vi "JsonTesting.vi"() -> ()   [LabVIEW 2012]
uses:
  <vilib>/httpClient/LabVIEWHTTPClient.lvlib
  <vilib>/LVH/i3 JSON/i3-json.lvlib
panel:
  out "body 3":string
  out "Tree 3":string(tree)
  out "body 2":string
  out "Tree 2":string(tree)
  out "Tree":string(tree)
  out "body":string
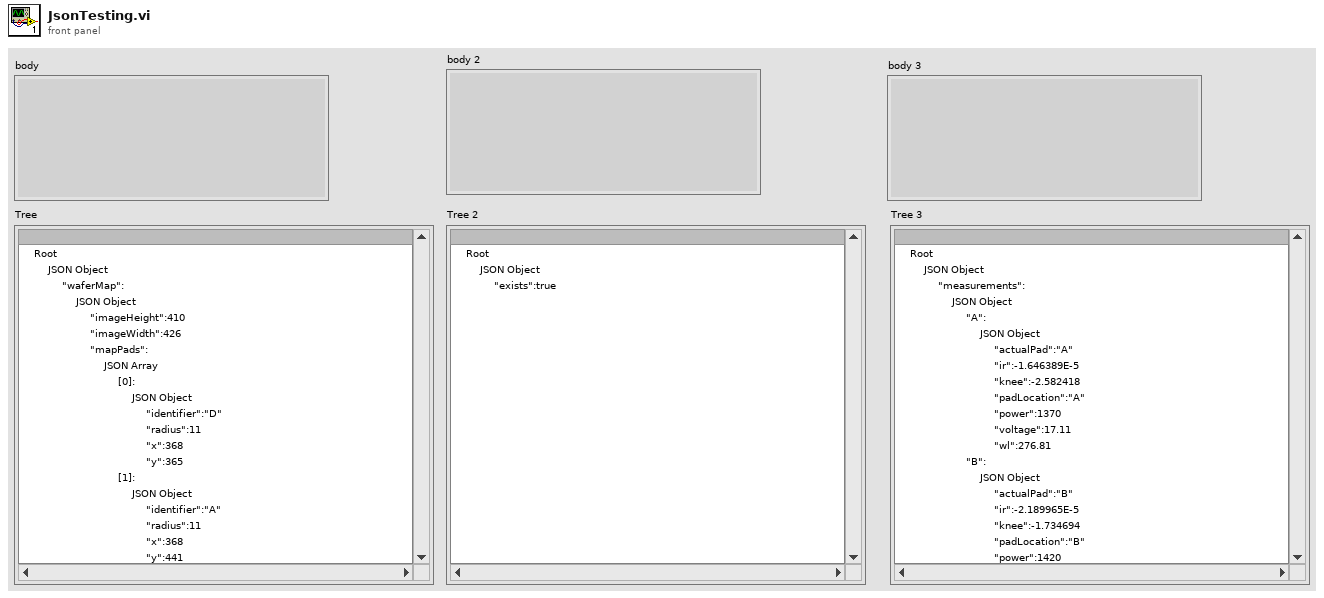
[diagram p1: front panel]
types:
  T1 = typedef "LabVIEWHTTPClient.lvlib/ClientHandle.ctl" = refnum<k1>
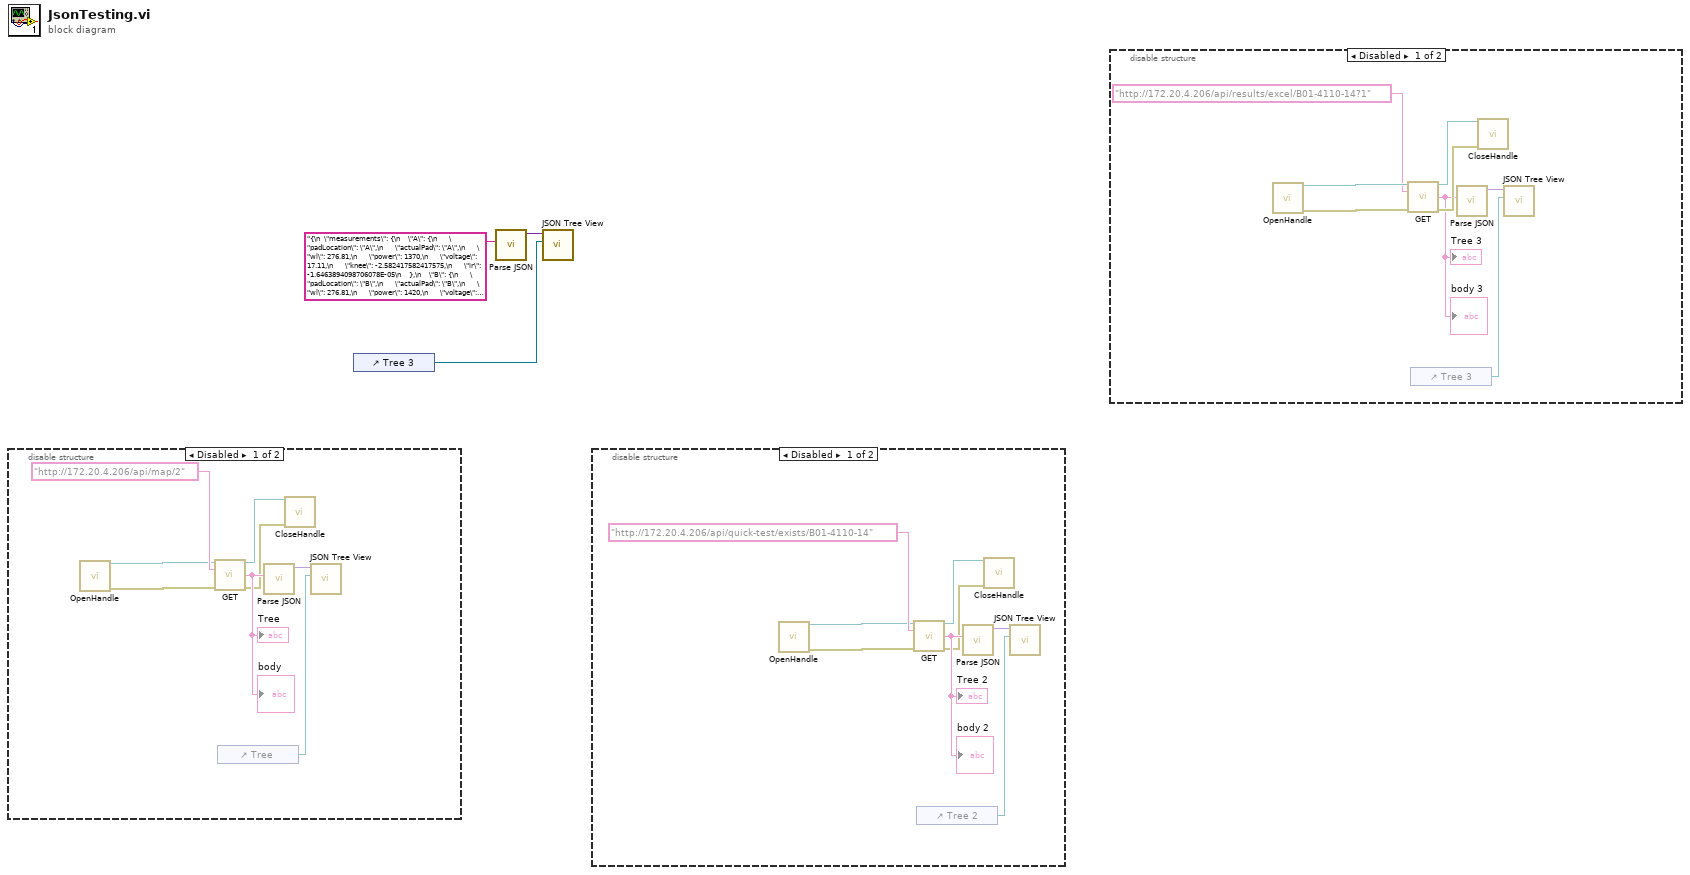
[diagram p0: block diagram]
diagram:
  n1 = disable-structure shown="Disabled" {
    frame Disabled {
      n2 = call <vilib>:"OpenHandle.vi"() -> ("client handle out"=w10:T1, "error out"=w9:errorcluster)  [unwired: 14 in]
      n3 = call <vilib>:"GET.vi"("client handle"=w10, "url"="http://172.20.4.206/api/map/2", "error in (no error)"=w9) -> ("client handle out"=w5:T1, "body"=w8:string, "error out"=w4:errorcluster)  [unwired: 9 in, 1 out]
      "body" <- w8
      "Tree" <- w8
      n4 = control-ref of="Tree"() -> (w6:refnum<vi>)
      n5 = call <vilib>:"Parse JSON.vi"("JSON String"=w8) -> ("JSON Tree"=w7:variant)  [unwired: 7 in, 3 out]
      n6 = call <vilib>:"CloseHandle.vi"("client handle"=w5, "error in (no error)"=w4) -> ()  [unwired: 13 in, 1 out]
      n7 = call <vilib>:"JSON Tree View.vi"("JSON Tree Expanded Reference"=w6, "JSON Tree"=w7) -> ()  [unwired: 8 in, 2 out]
    }
    frame Enabled {
    }
  }
  n8 = control-ref of="Tree 3"() -> (w1:refnum<vi>)
  n9 = call <vilib>:"Parse JSON.vi"("JSON String"="{\n  \"measurements\": {\n    \"A\": {\n      \"padLocation\": \"A\",\n      \"actualPad\": \"A\",\n      \"wl\": 276.81,\n      \"power\": 1370,\n      \"voltage\": 17.11,\n      \"knee\": -2.582417582417575,\n      \"ir\": -1.6463894098706078E-05\n    },\n    \"B\": {\n      \"padLocation\": \"B\",\n      \"actualPad\": \"B\",\n      \"wl\": 276.81,\n      \"power\": 1420,\n      \"voltage\": 17.28,\n      \"knee\": -1.7346938775510032,\n      \"ir\": -2.189965234720148E-05\n    },\n    \"C\": {\n      \"padLocation\": \"C\",\n      \"actualPad\": \"\",\n      \"wl\": 0,\n      \"power\": 0,\n      \"voltage\": 0,\n      \"knee\": 0,\n      \"ir\": 0\n    },\n    \"D\": {\n      \"padLocation\": \"D\",\n      \"actualPad\": \"\",\n      \"wl\": 0,\n      \"power\": 0,\n      \"voltage\": 0,\n      \"knee\": 0,\n      \"ir\": 0\n    },\n    \"G\": {\n      \"padLocation\": \"G\",\n      \"actualPad\": \"G2-E\",\n      \"wl\": 272.69,\n      \"power\": 1180,\n      \"voltage\": 15.45,\n      \"knee\": -0.7017543859649122,\n      \"ir\": -1.9614652410382404E-05\n    },\n    \"L\": {\n      \"padLocation\": \"L\",\n      \"actualPad\": \"L2-E\",\n      \"wl\": 273.81,\n      \"power\": 1310,\n      \"voltage\": 18.7,\n      \"knee\": -1.712707182320442,\n      \"ir\": -1.8277976050740107E-05\n    },\n    \"R\": {\n      \"padLocation\": \"R\",\n      \"actualPad\": \"R2-E\",\n      \"wl\": 274.94,\n      \"power\": 1270,\n      \"voltage\": 18.69,\n      \"knee\": -1.16666666666666,\n      \"ir\": -1.6391380995628424E-05\n    },\n    \"T\": {\n      \"padLocation\": \"T\",\n      \"actualPad\": \"T2-E\",\n      \"wl\": 274.94,\n      \"power\": 1290,\n      \"voltage\": 19.78,\n      \"knee\": -2.1142857142856957,\n      \"ir\": -1.2373818026389927E-05\n    }\n  }\n}") -> ("JSON Tree"=w3:variant)  [unwired: 7 in, 3 out]
  n10 = call <vilib>:"JSON Tree View.vi"("JSON Tree Expanded Reference"=w1, "JSON Tree"=w3) -> ()  [unwired: 8 in, 2 out]
  n11 = disable-structure shown="Disabled" {
    frame Disabled {
      n12 = call <vilib>:"OpenHandle.vi"() -> ("client handle out"=w18:T1, "error out"=w17:errorcluster)  [unwired: 14 in]
      n13 = call <vilib>:"GET.vi"("client handle"=w18, "url"="http://172.20.4.206/api/quick-test/exists/B01-4110-14", "error in (no error)"=w17) -> ("client handle out"=w13:T1, "body"=w16:string, "error out"=w12:errorcluster)  [unwired: 9 in, 1 out]
      "body 2" <- w16
      "Tree 2" <- w16
      n14 = control-ref of="Tree 2"() -> (w14:refnum<vi>)
      n15 = call <vilib>:"Parse JSON.vi"("JSON String"=w16) -> ("JSON Tree"=w15:variant)  [unwired: 7 in, 3 out]
      n16 = call <vilib>:"CloseHandle.vi"("client handle"=w13, "error in (no error)"=w12) -> ()  [unwired: 13 in, 1 out]
      n17 = call <vilib>:"JSON Tree View.vi"("JSON Tree Expanded Reference"=w14, "JSON Tree"=w15) -> ()  [unwired: 8 in, 2 out]
    }
    frame Enabled {
    }
  }
  n18 = disable-structure shown="Disabled" {
    frame Disabled {
      n19 = call <vilib>:"OpenHandle.vi"() -> ("client handle out"=w21:T1, "error out"=w22:errorcluster)  [unwired: 14 in]
      n20 = call <vilib>:"GET.vi"("client handle"=w21, "url"="http://172.20.4.206/api/results/excel/B01-4110-14?1", "error in (no error)"=w22) -> ("client handle out"=w26:T1, "body"=w23:string, "error out"=w27:errorcluster)  [unwired: 9 in, 1 out]
      "body 3" <- w23
      "Tree 3" <- w23
      n21 = control-ref of="Tree 3"() -> (w25:refnum<vi>)
      n22 = call <vilib>:"Parse JSON.vi"("JSON String"=w23) -> ("JSON Tree"=w24:variant)  [unwired: 7 in, 3 out]
      n23 = call <vilib>:"CloseHandle.vi"("client handle"=w26, "error in (no error)"=w27) -> ()  [unwired: 13 in, 1 out]
      n24 = call <vilib>:"JSON Tree View.vi"("JSON Tree Expanded Reference"=w25, "JSON Tree"=w24) -> ()  [unwired: 8 in, 2 out]
    }
    frame Enabled {
    }
  }
